vi "采集.vi"() -> (3 "Data":T1)   [LabVIEW 2019]
uses:
  <userlib>/DAQNavi Polymorphic VI/create/DAQNavi Create Channel(AI-Voltage).vi
  <userlib>/DAQNavi Polymorphic VI/configure/timing/DAQNavi Timing(AI Convert Clock).vi
  <userlib>/DAQNavi Polymorphic VI/read/DAQNavi Read (Analog 1D DBL NChan 1Samp).vi
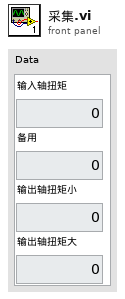
[diagram p1: front panel]
types:
  T1 = cluster{"输入轴扭矩":dbl, "备用":dbl, "输出轴扭矩小":dbl, "输出轴扭矩大":dbl}
  T2 = cluster{"[0]":dbl, "[1]":dbl, "[2]":dbl, "[3]":dbl}
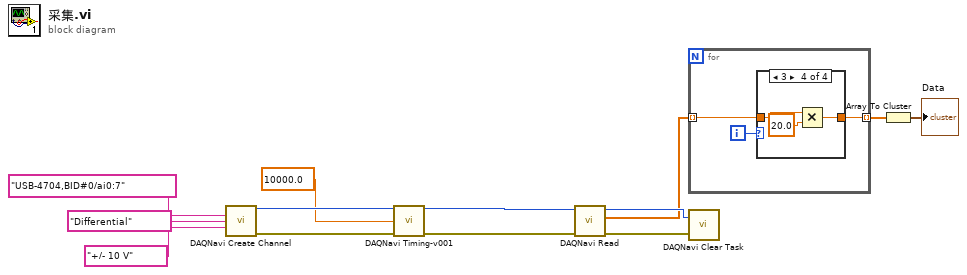
[diagram p0: block diagram]
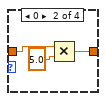
[diagram p3: hidden frame]
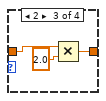
[diagram p4: hidden frame]
diagram:
  n1 = call-poly <userlib>:"DAQNavi Create Channel.vi"("physical channels"="USB-4704,BID#0/ai0:7", "signal type"="Differential", "value range"="+/- 10 V") -> ("task out"=w11:i32, "error out"=w9:errorcluster)  [unwired: 11 in]
  n2 = call-poly <userlib>:"DAQNavi Timing-v001.vi"("task in"=w11, "rate"=10000.0, "error in (no error)"=w9) -> ("task out"=w10:i32, "error out"=w8:errorcluster)  [unwired: 11 in]
  n3 = call-poly <userlib>:"DAQNavi Read.vi"("error in (no error)"=w8, "task in"=w10) -> ("error out"=w4:errorcluster, "data"=w2:dbl[], "task out"=w5:i32)  [unwired: 7 in]
  n4 = for {
    tunnel: w2 -> [w15] mode=indexing
    tunnel: [w14] -> w1 mode=indexing
    i -> [w16]
    n5 = case shown="3" w16 {
      tunnel: w15 -> [w17 w20 w23 w26]
      tunnel: [w17 w18 w21 w24] -> w14
      frame 1, Default {
      }
      frame 0 {
        n6 = Multiply(x=w20, y=5.0) -> (x*y=w18:dbl)
      }
      frame 2 {
        n7 = Multiply(x=w23, y=2.0) -> (x*y=w21:dbl)
      }
      frame 3 {
        n8 = Multiply(x=w26, y=20.0) -> (x*y=w24:dbl)
      }
    }
  }
  n9 = call <userlib>:"DAQNavi Clear Task.vi"("error in (no error)"=w4, "task in"=w5) -> ()  [unwired: 1 in, 1 out]
  n10 = Array To Cluster(array=w1) -> (cluster=→"Data":T2)
